vi "Labview_USB_SPI_W25Q32.vi"() -> ()   [LabVIEW 2010]
uses:
  <userlib>/Ginkgo_Driver/Ginkgo_Driver.dll
panel:
  out "Flag(T:read;F:write)":bool=TRUE
  in  "pInitConfig":T1
  in  "Constant":T2={"DevType"=1, "DevIndex"=0, "SPIIndex"=0, "Addr"=0, "SubAddr"=0}
  out "error out":errorcluster
  in  "Slave Addr(Hex)":u8 format="%x"
  in  "Sub Addr(Hex)":u8 format="%x"
  in  "Read":bool
  in  "Write":bool
  out "Read Data(Hex)":string
  in  "Write Data(Hex)":string
  in  "Channel Index":u16(ring) items=["0", "1"]
  in  "Speed":u32(ring)=36000000 items=["36000Kbps"=36000000, "18000Kbps"=18000000, "9000Kbps"=9000000, "4500Kbps"=4500000, "2250Kbps"=2250000]
  in  "Device Index":u16(ring) items=["0", "1", "2", "3", "4", "5", "6", "7", "8", "9"]
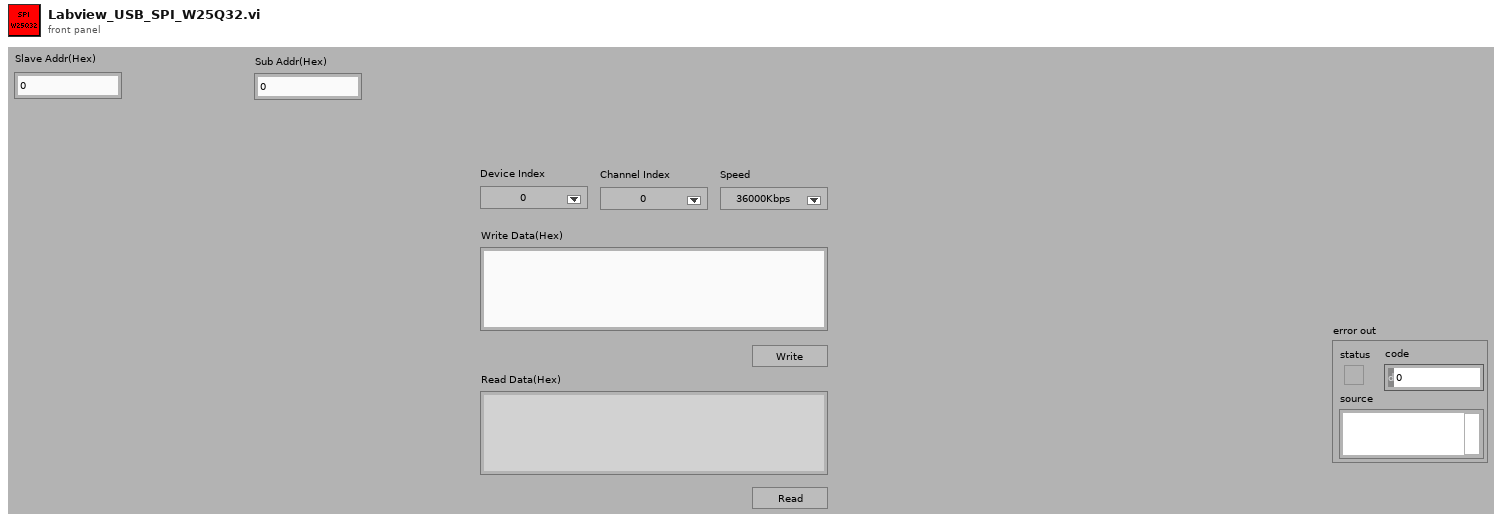
[diagram p1: front panel]
types:
  T1 = cluster{"ControlMode":u8, "TranBits":u8, "MasterMode":u8, "CPOL":u8, "CPHA":u8, "LSBFirst":u8, "SelPolarity":u8, "@dummy control@":i8, "ClockSpeed":u32}
  T2 = cluster{"DevType":i32, "DevIndex":i32, "SPIIndex":i32, "Addr":u16, "SubAddr":u32}
  T3 = enum16{"Init", "Write", "Read", "Idel", "Close", "Error"}
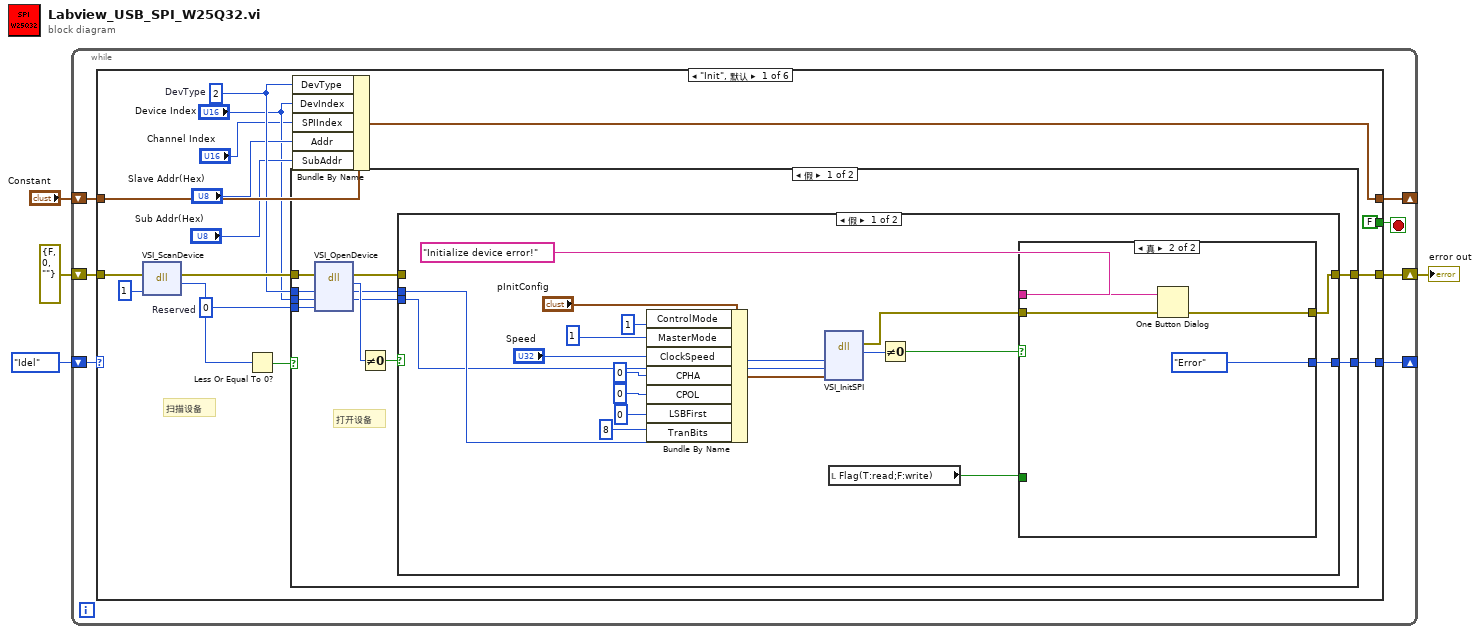
[diagram p0: block diagram]
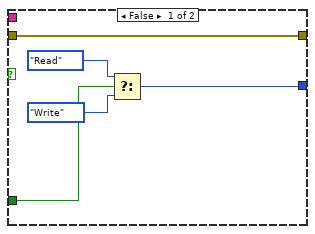
[diagram p2: hidden frame]
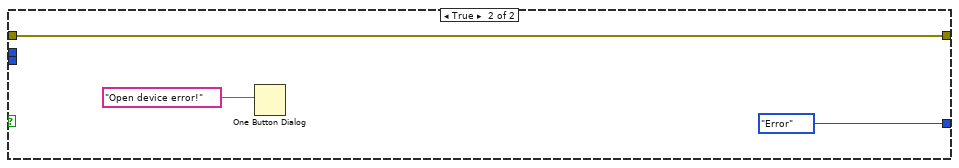
[diagram p3: hidden frame]
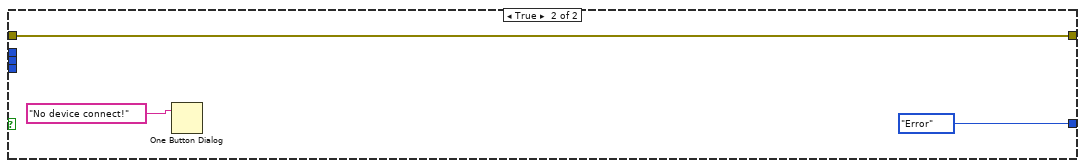
[diagram p4: hidden frame]
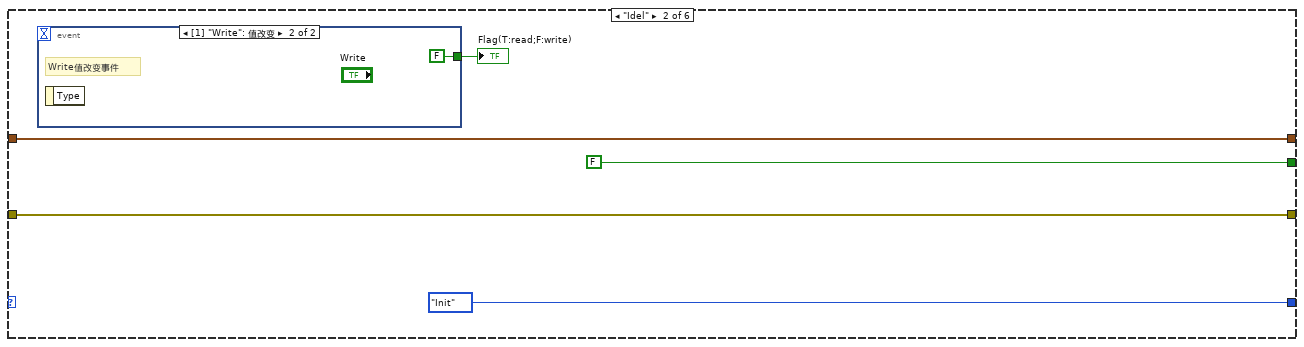
[diagram p5: hidden frame]
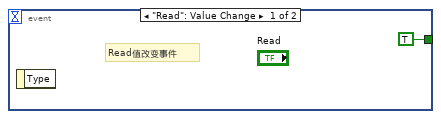
[diagram p6: hidden frame]
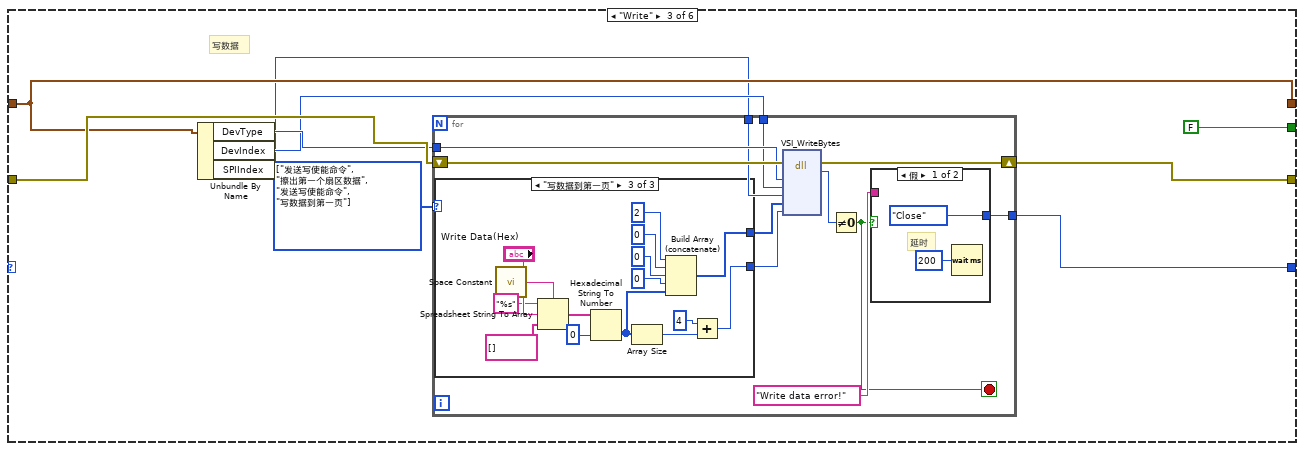
[diagram p7: hidden frame]
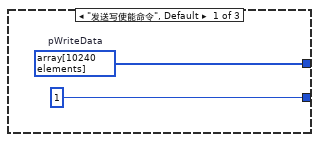
[diagram p8: hidden frame]
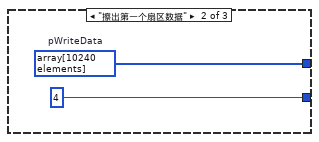
[diagram p9: hidden frame]
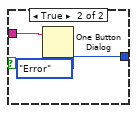
[diagram p10: hidden frame]
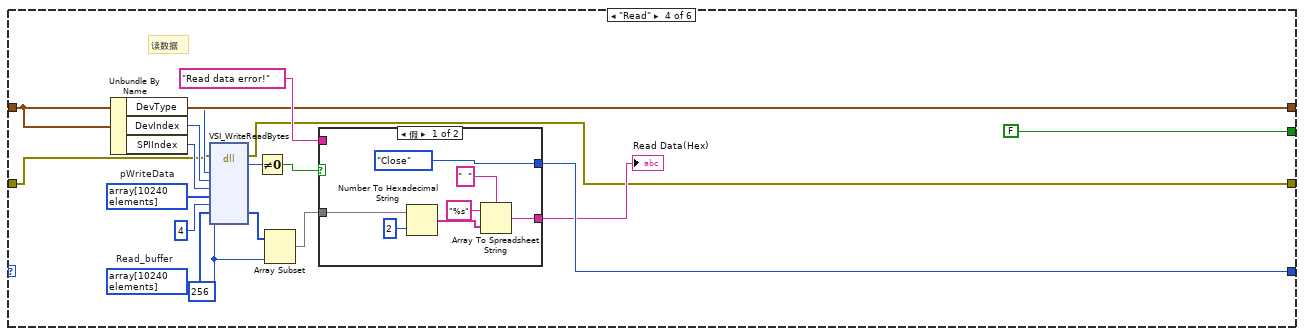
[diagram p11: hidden frame]
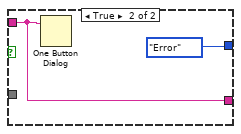
[diagram p12: hidden frame]
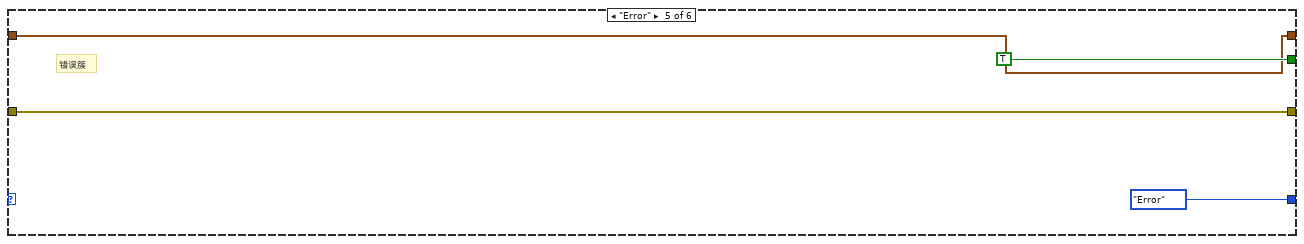
[diagram p13: hidden frame]
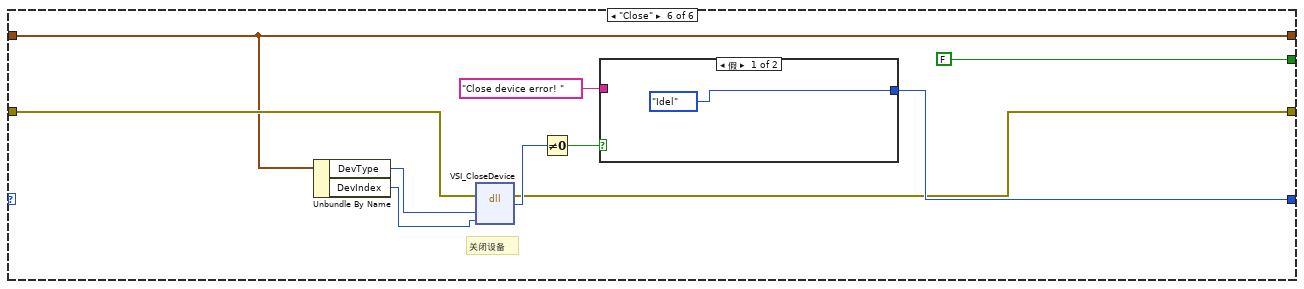
[diagram p14: hidden frame]
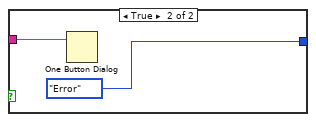
[diagram p15: hidden frame]
diagram:
  n1 = while {
    shift-right: [w11] -> _
    shift-left: T3."Idel" ("Enum") -> [w10]
    shift-right: [w8] -> w2
    shift-left: errorcluster {"status"=FALSE, "code"=0, "source"=""} ("error out") -> [w7]
    shift-right: [w5] -> _
    shift-left: "Constant" -> [w6]
    stop <- w9 stop-if-true
    n2 = case shown="\"Init\", 默认" w10 {
      tunnel: [w19 T3."Init" ("Enum") w78 w137 T3."Error" ("Enum") w158] -> w11
      tunnel: [FALSE ("stop") FALSE ("stop") FALSE ("stop") FALSE ("stop") TRUE ("stop") FALSE ("stop")] -> w9
      tunnel: [w20 w74 w79 w128 w151 w157] -> w8
      tunnel: w7 -> [w21 w74 w84 w130 w151 w156]
      tunnel: w6 -> [w18 w73 w83 w136 w149 w155]
      tunnel: [w14 w73 w83 w136 w149 w155] -> w5
      frame "Init", Default {
        w22 = 0  # Reserved
        w17 = 2  # DevType
        # "扫描设备"
        n3 = dll-call lib="D:/Program Files (x86)/National Instruments/LabVIEW 2010/user.lib/Ginkgo_Driver/Ginkgo_Driver.*" fn="VSI_ScanDevice"(error in=w21, "NeedInit"=u8 1) -> (error out=w23:errorcluster, "return type"=w25:i32)  [unwired: 3 in, 1 out]
        n4 = Less Or Equal To 0?(x=w25) -> (x <= 0?=w24:bool)
        n5 = case shown="假" w24 {
          tunnel: [w32 T3."Error" ("Enum")] -> w19
          tunnel: w23 -> [w36 w69]
          tunnel: w22 -> [w35 _]
          tunnel: "Device Index" -> [w34 _]
          tunnel: w17 -> [w33 _]
          tunnel: [w28 w69] -> w20
          frame False {
            # "打开设备"
            n6 = dll-call lib="D:/Program Files (x86)/National Instruments/LabVIEW 2010/user.lib/Ginkgo_Driver/Ginkgo_Driver.*" fn="VSI_OpenDevice"(error in=w36, "DevType"=w33, "DevIndex"=w34, "Reserved"=w35) -> (error out=w31:errorcluster, "return type"=w37:i32, "DevType"=w30:i32, "DevIndex"=w29:i32)  [unwired: 3 in, 1 out]
            n7 = Not Equal To 0?(x=w37) -> (x != 0?=w38:bool)
            n8 = case shown="假" w38 {
              tunnel: [w53 T3."Error" ("Enum")] -> w32
              tunnel: w31 -> [_ w66]
              tunnel: w30 -> [w47 _]
              tunnel: w29 -> [w46 _]
              tunnel: [w52 w66] -> w28
              frame False {
                n9 = Bundle By Name(cluster="pInitConfig", "ControlMode"=u8 1 ("AddrType"), "MasterMode"=u8 1 ("SubAddrWidth"), "ClockSpeed"="Speed", "CPHA"=u8 0 ("ControlMode"), "CPOL"=u8 0 ("MasterMode"), "LSBFirst"=u8 0, "TranBits"=u8 8) -> (w42:T1)
                n10 = dll-call lib="D:/Program Files (x86)/National Instruments/LabVIEW 2010/user.lib/Ginkgo_Driver/Ginkgo_Driver.*" fn="VSI_InitSPI"("DevType"=w47, "DevIndex"=w46, "pInitConfig"=w42) -> (error out=w40:errorcluster, w41:i32)  [unwired: 6 in, 1 out]
                n11 = local read "Flag(T:read;F:write)"() -> (w39:bool)
                n12 = Not Equal To 0?(x=w41) -> (x != 0?=w56:bool)
                n13 = case shown="真" w56 {
                  tunnel: "Initialize device error!" ("message") -> [_ w64]
                  tunnel: [w59 T3."Error" ("Enum")] -> w53
                  tunnel: w40 -> [w58 w62]
                  tunnel: [w58 w62] -> w52
                  tunnel: w39 -> [w57 _]
                  frame False {
                    n14 = Select(t=T3."Read" ("Enum"), s=w57, f=T3."Write" ("Enum")) -> (s? t:f=w59:T3)
                  }
                  frame True {
                    n15 = One Button Dialog(message=w64) -> ()  [unwired: 1 in, 1 out]
                  }
                }
              }
              frame True {
                n16 = One Button Dialog(message="Open device error!") -> ()  [unwired: 1 in, 1 out]
              }
            }
          }
          frame True {
            n17 = One Button Dialog(message="No device connect!") -> ()  [unwired: 1 in, 1 out]
          }
        }
        n18 = Bundle By Name(cluster=w18, "DevType"=w17, "DevIndex"="Device Index", "SPIIndex"="Channel Index", "Addr"="Slave Addr(Hex)", "SubAddr"="Sub Addr(Hex)") -> (w14:T2)
      }
      frame "Idel" {
        n19 = event shown="[1] \"Write\": 值改变" {
          selector: _ -> [_ _]
          dyn-events: _ -> [_ _]
          timeout: _ -> [_ _]
          tunnel: [TRUE FALSE] -> w72
          event "Read": Value Change {
            # "Read值改变事件"
            n20 = event-data() -> ()  [unwired: 1 in, 1 out]
          }
          event "Write": Value Change {
            # "Write值改变事件"
            n21 = event-data() -> ()  [unwired: 1 in, 1 out]
          }
        }
        "Flag(T:read;F:write)" <- w72
      }
      frame "Write" {
        w85 = enum16{"发送写使能命令", "擦出第一个扇区数据", "写数据到第一页"}[] [enum."发送写使能命令", enum."擦出第一个扇区数据", enum."发送写使能命令", enum."写数据到第一页"] items=["发送写使能命令", "擦出第一个扇区数据", "写数据到第一页"]
        # "写数据"
        n22 = Unbundle By Name(w83) -> ("DevType"=w82:i32, "DevIndex"=w81:i32, "SPIIndex"=w80:i32)
        n23 = for {
          tunnel: w85 -> [w94] mode=indexing
          shift-right: [w93] -> w79
          shift-left: w84 -> [w92]
          tunnel: [w91] -> w78
          tunnel: w82 -> [w90]
          tunnel: w81 -> [w89]
          tunnel: w80 -> [w88]
          stop <- w87 stop-if-true
          n24 = case shown="\"写数据到第一页\"" w94 {
            tunnel: [w100 w101 w111] -> w96
            tunnel: [u16 1 ("Len") u16 4 ("Len") w116] -> w95
            frame "发送写使能命令", Default {
              w100 = u8[] array[10240 elements]  # pWriteData
            }
            frame "擦出第一个扇区数据" {
              w101 = u8[] array[10240 elements]  # pWriteData
            }
            frame "写数据到第一页" {
              n25 = call <vilib>:"Space Constant.vi"() -> ("String"=w104:string)
              n26 = Spreadsheet String To Array(delimiter (Tab)=w104, format string="%s", spreadsheet string="Write Data(Hex)", array type (2D Dbl)=string[] []) -> (array=w107:string[])
              n27 = Hexadecimal String To Number(string=w107, default (0uL)=u8 0 ("default (0 U32)")) -> (number=w103:u8[])  [unwired: 1 in, 1 out]
              n28 = Array Size(array=w103) -> (size(s)=w110:i32)
              n29 = Build Array (concatenate)(u8 2 ("数值"), u8 0 ("数值"), u8 0 ("数值"), u8 0 ("数值"), w103) -> (w111:u8[])
              n30 = Add(x=u16 4, y=w110) -> (x+y=w116:i32)
            }
          }
          n31 = dll-call lib="D:/Program Files (x86)/National Instruments/LabVIEW 2010/user.lib/Ginkgo_Driver/Ginkgo_Driver.*" fn="VSI_WriteBytes"(error in=w92, "DevType"=w90, "DevIndex"=w89, "SPIIndex"=w88, "pWriteData"=w96, "Len"=w95) -> (error out=w93:errorcluster, w97:i32)  [unwired: 7 in, 1 out]
          n32 = Not Equal To 0?(x=w97) -> (x != 0?=w87:bool)
          n33 = case shown="假" w87 {
            tunnel: "Write data error!" ("message") -> [_ w121]
            tunnel: [T3."Close" ("Enum") T3."Error" ("Enum")] -> w91
            frame False {
              # "延时"
              n34 = Wait (ms)(milliseconds to wait=u32 200) -> ()  [unwired: 1 out]
            }
            frame True {
              n35 = One Button Dialog(message=w121) -> ()  [unwired: 1 in, 1 out]
            }
          }
        }
      }
      frame "Read" {
        w124 = u16 256 ("ReadLen")
        w125 = u8[] array[10240 elements]  # pWriteData
        w127 = u8[] array[10240 elements]  # Read_buffer
        # "读数据"
        n36 = Unbundle By Name(w136) -> ("DevType"=w133:i32, "DevIndex"=w132:i32, "SPIIndex"=w131:i32)
        n37 = dll-call lib="D:/Program Files (x86)/National Instruments/LabVIEW 2010/user.lib/Ginkgo_Driver/Ginkgo_Driver.*" fn="VSI_WriteReadBytes"(error in=w130, "DevType"=w133, "DevIndex"=w132, "SPIIndex"=w131, "pWriteData"=w125, "WriteLen"=u16 4, "pReadData"=w127, "ReadLen"=w124) -> (error out=w128:errorcluster, w129:i32, "pReadData"=w123:u8[])  [unwired: 8 in, 1 out]
        n38 = Not Equal To 0?(x=w129) -> (x != 0?=w135:bool)
        n39 = Array Subset(array=w123, length=w124) -> (w122:u8[])  [unwired: 1 in]
        n40 = case shown="假" w135 {
          tunnel: "Read data error!" ("message") -> [_ w147]
          tunnel: [T3."Close" ("Enum") T3."Error" ("Enum")] -> w137
          tunnel: w122 -> [w141 _]
          tunnel: [w140 w147] -> w134
          frame False {
            n41 = Number To Hexadecimal String(1:i16 2 ("width (-)"), 2:w141) -> (0:w143:string[])
            n42 = Array To Spreadsheet String(delimiter (Tab)="  ", array=w143, 3:"%s" ("format string")) -> (spreadsheet string=w140:string)
          }
          frame True {
            n43 = One Button Dialog(message=w147) -> ()  [unwired: 1 in, 1 out]
          }
        }
        "Read Data(Hex)" <- w134
      }
      frame "Error" {
        # "错误簇"
      }
      frame "Close" {
        # "关闭设备"
        n44 = Unbundle By Name(w155) -> ("DevType"=w154:i32, "DevIndex"=w153:i32)
        n45 = dll-call lib="D:/Program Files (x86)/National Instruments/LabVIEW 2010/user.lib/Ginkgo_Driver/Ginkgo_Driver.*" fn="VSI_CloseDevice"(error in=w156, "DevType"=w154, "DevIndex"=w153) -> (error out=w157:errorcluster, "return type"=w160:i32)  [unwired: 4 in, 1 out]
        n46 = Not Equal To 0?(x=w160) -> (x != 0?=w159:bool)
        n47 = case shown="假" w159 {
          tunnel: "Close device error! " ("message") -> [_ w165]
          tunnel: [T3."Idel" ("Enum") T3."Error" ("Enum")] -> w158
          frame False {
          }
          frame True {
            n48 = One Button Dialog(message=w165) -> ()  [unwired: 1 in, 1 out]
          }
        }
      }
    }
  }
  "error out" <- w2
